vi "main.vi"() -> ()   [LabVIEW 2023]
uses:
  #typedef_state.ctl
  #typedef_action.ctl
  #typedef_data.ctl
panel:
  in  "Mode":dbl(knob) scale=0.0..4.0
  in  "Lid Open 2":bool
  in  "Drying Enable":bool
  in  "Start":bool
  in  "stop":bool
  out "Lid Open":bool
  out "Drying":bool
  out "Centrifugation":bool
  out "Pump watter out":bool
  out "Motor controll":bool
  out "Water heating":bool
  out "Power ON":bool
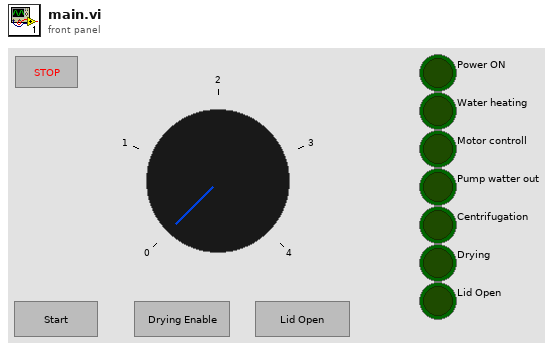
[diagram p1: front panel]
types:
  T1 = typedef "#typedef_state.ctl" = enum16{"Stop", "Drying", "Centrifugation", "Pump watter out", "Motor controll", "Water heating", "Idling", "Inicializing"}
  T2 = typedef "#typedef_action.ctl" = enum16{"pause", "reset", "run"}
  T3 = enum8{"Enabled", "Disabled", "Disabled and Grayed Out"}
  T4 = typedef "#typedef_data.ctl" = cluster{"Power ON":bool, "Water heating":bool, "Motor controll":bool, "Pump watter out":bool, "Centrifugation":bool, "Drying":bool, "Lid Open":bool, "stop":bool, "Start":bool, "Drying Enable":bool, "Lid Open 2":bool, "Mode":dbl, "timereset?":bool}
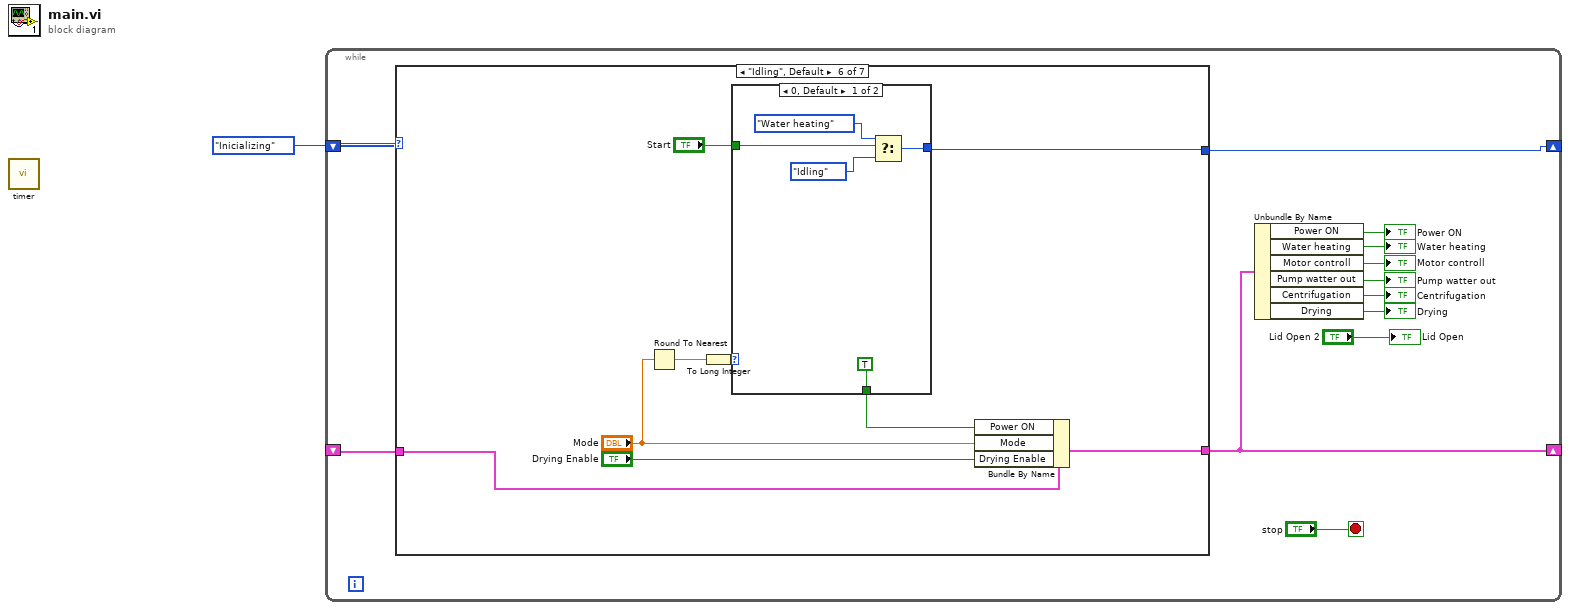
[diagram p0: block diagram]
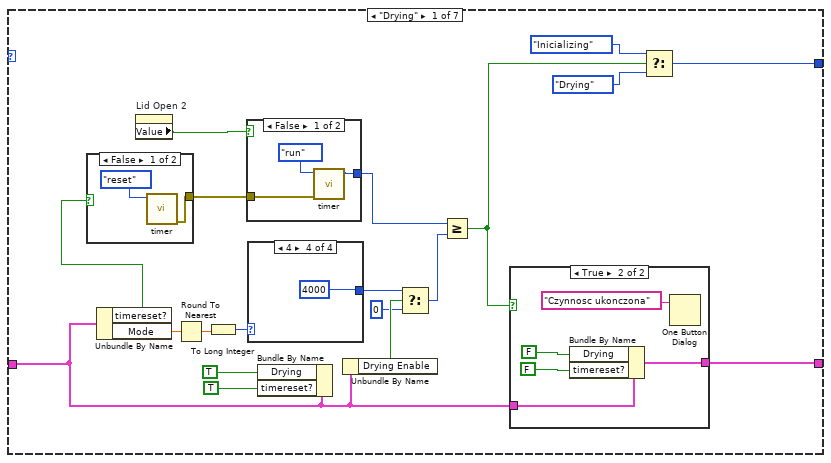
[diagram p2: hidden frame]
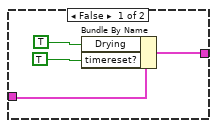
[diagram p3: hidden frame]
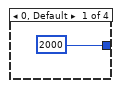
[diagram p4: hidden frame]
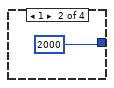
[diagram p5: hidden frame]
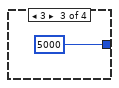
[diagram p6: hidden frame]
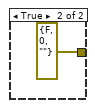
[diagram p7: hidden frame]
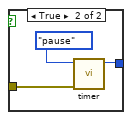
[diagram p8: hidden frame]
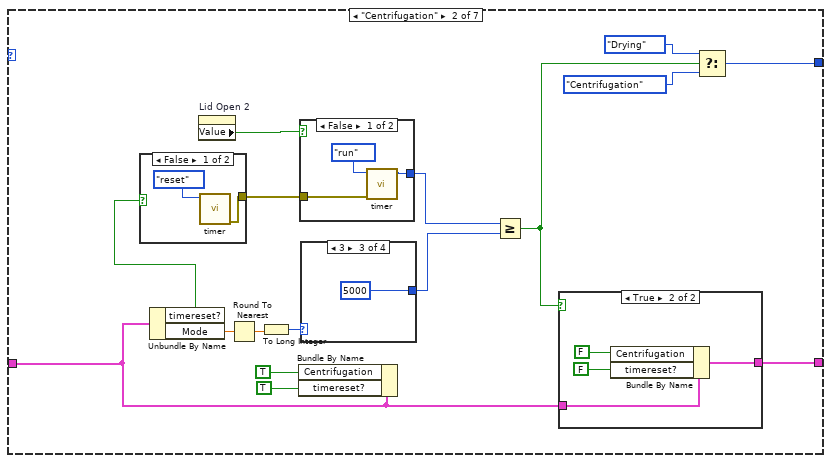
[diagram p9: hidden frame]
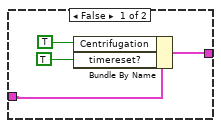
[diagram p10: hidden frame]
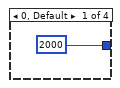
[diagram p11: hidden frame]
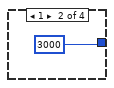
[diagram p12: hidden frame]
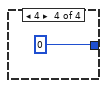
[diagram p13: hidden frame]
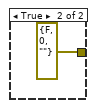
[diagram p14: hidden frame]
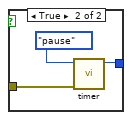
[diagram p15: hidden frame]
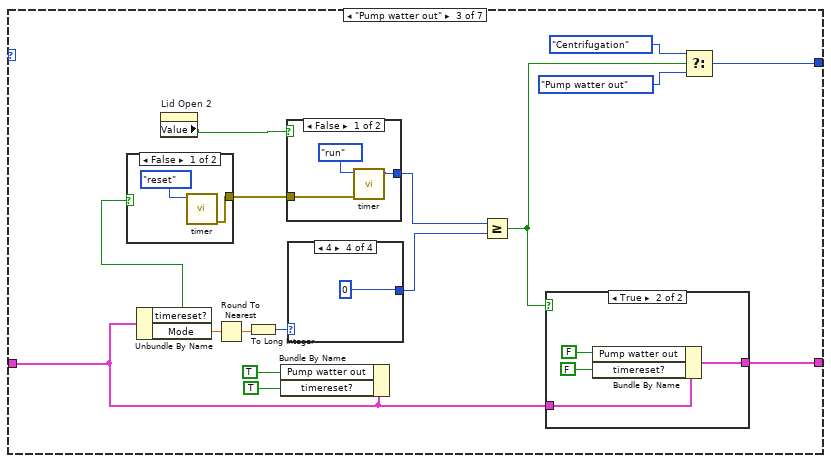
[diagram p16: hidden frame]
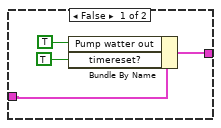
[diagram p17: hidden frame]
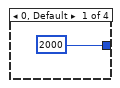
[diagram p18: hidden frame]
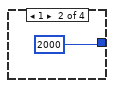
[diagram p19: hidden frame]
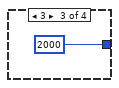
[diagram p20: hidden frame]
diagram:
  n1 = call "timer.vi"() -> ()  [unwired: 10 in, 2 out]
  n2 = while {
    shift-right: [w11] -> _
    shift-left: #typedef_state."Inicializing" ("State") -> [w13]
    shift-right: [w10] -> _
    shift-left: _ -> [w12]
    stop <- "stop" stop-if-true
    n3 = case shown="\"Idling\", Default" w13 {
      tunnel: [w20 w55 w93 w132 w170 w212 T4 {"Power ON"=FALSE, "Water heating"=FALSE, "Motor controll"=FALSE, "Pump watter out"=FALSE, "Centrifugation"=FALSE, "Drying"=FALSE, "Lid Open"=FALSE, "stop"=FALSE, "Start"=FALSE, "Drying Enable"=FALSE, "Lid Open 2"=FALSE, "Mode"=2.05168848812912, "timereset?"=FALSE} ("Data")] -> w10
      tunnel: w12 -> [w18 w56 w94 w131 w171 w213 _]
      tunnel: [w19 w57 w92 w129 w168 w206 #typedef_state."Idling" ("State")] -> w11
      frame "Drying" {
        n4 = Unbundle By Name(w18) -> ("timereset?"=w32:bool, "Mode"=w30:dbl)
        n5 = case shown="False" w32 {
          tunnel: [w46 errorcluster {"status"=FALSE, "code"=0, "source"=""} ("error out")] -> w31
          frame False {
            n6 = call "timer.vi"("Action"=#typedef_action."reset") -> ("error out"=w46:errorcluster)  [unwired: 9 in, 1 out]
          }
          frame True {
          }
        }
        n7 = property on="Lid Open 2" class="Bool (strict)"() -> ("Value"=w21:bool)  [unwired: 2 in, 2 out]
        n8 = Round To Nearest(number=w30) -> (nearest integer value=w26:dbl)
        n9 = To Long Integer(number=w26) -> (32bit integer=w27:i32)
        n10 = case shown="False" w21 {
          tunnel: w31 -> [w51 w53]
          tunnel: [w49 w52] -> w25
          frame False {
            n11 = call "timer.vi"("error in (no error)"=w51, "Action"=#typedef_action."run") -> ("Numeric"=w49:u32)  [unwired: 8 in, 1 out]
          }
          frame True {
            n12 = call "timer.vi"("error in (no error)"=w53, "Action"=#typedef_action."pause") -> ("Numeric"=w52:u32)  [unwired: 8 in, 1 out]
          }
        }
        n13 = case shown="4" w27 {
          tunnel: [2000 2000 5000 4000] -> w15
          frame 0, Default {
          }
          frame 1 {
          }
          frame 3 {
          }
          frame 4 {
          }
        }
        n14 = Bundle By Name(cluster=w18, "Drying"=TRUE ("Water heating"), "timereset?"=TRUE) -> ()  [unwired: 1 out]
        n15 = Unbundle By Name(w18) -> ("Drying Enable"=w17:bool)
        n16 = Select(t=w15, s=w17, f=0) -> (s? t:f=w14:i32)
        n17 = Greater Or Equal?(x=w25, y=w14) -> (x >= y?=w24:bool)
        n18 = case shown="True" w24 {
          tunnel: w18 -> [w33 w39]
          tunnel: [w34 w38] -> w20
          frame False {
            n19 = Bundle By Name(cluster=w33, "Drying"=TRUE ("Water heating"), "timereset?"=TRUE) -> (w34:T4)
          }
          frame True {
            n20 = Bundle By Name(cluster=w39, "Drying"=FALSE ("Water heating"), "timereset?"=FALSE) -> (w38:T4)
            n21 = One Button Dialog(message="Czynnosc ukonczona") -> ()  [unwired: 1 in, 1 out]
          }
        }
        n22 = Select(t=#typedef_state."Inicializing" ("State"), s=w24, f=#typedef_state."Drying") -> (s? t:f=w19:T1)
      }
      frame "Centrifugation" {
        n23 = Unbundle By Name(w56) -> ("timereset?"=w70:bool, "Mode"=w68:dbl)
        n24 = case shown="False" w70 {
          tunnel: [w83 errorcluster {"status"=FALSE, "code"=0, "source"=""} ("error out")] -> w69
          frame False {
            n25 = call "timer.vi"("Action"=#typedef_action."reset") -> ("error out"=w83:errorcluster)  [unwired: 9 in, 1 out]
          }
          frame True {
          }
        }
        n26 = property on="Lid Open 2" class="Bool (strict)"() -> ("Value"=w58:bool)  [unwired: 2 in, 2 out]
        n27 = Round To Nearest(number=w68) -> (nearest integer value=w64:dbl)
        n28 = To Long Integer(number=w64) -> (32bit integer=w65:i32)
        n29 = Bundle By Name(cluster=w56, "Centrifugation"=TRUE ("Water heating"), "timereset?"=TRUE) -> ()  [unwired: 1 out]
        n30 = case shown="False" w58 {
          tunnel: w69 -> [w88 w90]
          tunnel: [w86 w89] -> w63
          frame False {
            n31 = call "timer.vi"("error in (no error)"=w88, "Action"=#typedef_action."run") -> ("Numeric"=w86:u32)  [unwired: 8 in, 1 out]
          }
          frame True {
            n32 = call "timer.vi"("error in (no error)"=w90, "Action"=#typedef_action."pause") -> ("Numeric"=w89:u32)  [unwired: 8 in, 1 out]
          }
        }
        n33 = case shown="3" w65 {
          tunnel: [2000 3000 5000 0] -> w62
          frame 0, Default {
          }
          frame 1 {
          }
          frame 3 {
          }
          frame 4 {
          }
        }
        n34 = Greater Or Equal?(x=w63, y=w62) -> (x >= y?=w61:bool)
        n35 = case shown="True" w61 {
          tunnel: w56 -> [w71 w76]
          tunnel: [w72 w75] -> w55
          frame False {
            n36 = Bundle By Name(cluster=w71, "Centrifugation"=TRUE ("Water heating"), "timereset?"=TRUE) -> (w72:T4)
          }
          frame True {
            n37 = Bundle By Name(cluster=w76, "Centrifugation"=FALSE ("Water heating"), "timereset?"=FALSE) -> (w75:T4)
          }
        }
        n38 = Select(t=#typedef_state."Drying" ("State"), s=w61, f=#typedef_state."Centrifugation") -> (s? t:f=w57:T1)
      }
      frame "Pump watter out" {
        n39 = Unbundle By Name(w94) -> ("timereset?"=w107:bool, "Mode"=w105:dbl)
        n40 = case shown="False" w107 {
          tunnel: [w120 errorcluster {"status"=FALSE, "code"=0, "source"=""} ("error out")] -> w106
          frame False {
            n41 = call "timer.vi"("Action"=#typedef_action."reset") -> ("error out"=w120:errorcluster)  [unwired: 9 in, 1 out]
          }
          frame True {
          }
        }
        n42 = property on="Lid Open 2" class="Bool (strict)"() -> ("Value"=w95:bool)  [unwired: 2 in, 2 out]
        n43 = Round To Nearest(number=w105) -> (nearest integer value=w101:dbl)
        n44 = To Long Integer(number=w101) -> (32bit integer=w102:i32)
        n45 = Bundle By Name(cluster=w94, "Pump watter out"=TRUE ("Water heating"), "timereset?"=TRUE) -> ()  [unwired: 1 out]
        n46 = case shown="False" w95 {
          tunnel: w106 -> [w125 w127]
          tunnel: [w123 w126] -> w100
          frame False {
            n47 = call "timer.vi"("error in (no error)"=w125, "Action"=#typedef_action."run") -> ("Numeric"=w123:u32)  [unwired: 8 in, 1 out]
          }
          frame True {
            n48 = call "timer.vi"("error in (no error)"=w127, "Action"=#typedef_action."pause") -> ("Numeric"=w126:u32)  [unwired: 8 in, 1 out]
          }
        }
        n49 = case shown="4" w102 {
          tunnel: [2000 2000 2000 0] -> w99
          frame 0, Default {
          }
          frame 1 {
          }
          frame 3 {
          }
          frame 4 {
          }
        }
        n50 = Greater Or Equal?(x=w100, y=w99) -> (x >= y?=w98:bool)
        n51 = case shown="True" w98 {
          tunnel: w94 -> [w108 w113]
          tunnel: [w109 w112] -> w93
          frame False {
            n52 = Bundle By Name(cluster=w108, "Pump watter out"=TRUE ("Water heating"), "timereset?"=TRUE) -> (w109:T4)
          }
          frame True {
            n53 = Bundle By Name(cluster=w113, "Pump watter out"=FALSE ("Water heating"), "timereset?"=FALSE) -> (w112:T4)
          }
        }
        n54 = Select(t=#typedef_state."Centrifugation" ("State"), s=w98, f=#typedef_state."Pump watter out") -> (s? t:f=w92:T1)
      }
      frame "Motor controll" {
        n55 = Unbundle By Name(w131) -> ("timereset?"=w144:bool, "Mode"=w142:dbl)
        n56 = case shown="False" w144 {
          tunnel: [w157 errorcluster {"status"=FALSE, "code"=0, "source"=""} ("error out")] -> w143
          frame False {
            n57 = call "timer.vi"("Action"=#typedef_action."reset") -> ("error out"=w157:errorcluster)  [unwired: 9 in, 1 out]
          }
          frame True {
          }
        }
        n58 = property on="Lid Open 2" class="Bool (strict)"() -> ("Value"=w130:bool)  [unwired: 2 in, 2 out]
        n59 = Round To Nearest(number=w142) -> (nearest integer value=w138:dbl)
        n60 = To Long Integer(number=w138) -> (32bit integer=w139:i32)
        n61 = case shown="False" w130 {
          tunnel: w143 -> [w162 w164]
          tunnel: [w160 w163] -> w137
          frame False {
            n62 = call "timer.vi"("error in (no error)"=w162, "Action"=#typedef_action."run") -> ("Numeric"=w160:u32)  [unwired: 8 in, 1 out]
          }
          frame True {
            n63 = call "timer.vi"("error in (no error)"=w164, "Action"=#typedef_action."pause") -> ("Numeric"=w163:u32)  [unwired: 8 in, 1 out]
          }
        }
        n64 = Bundle By Name(cluster=w131, "Motor controll"=TRUE ("Water heating"), "timereset?"=TRUE) -> ()  [unwired: 1 out]
        n65 = case shown="3" w139 {
          tunnel: [2000 4000 6000 0] -> w136
          frame 0, Default {
          }
          frame 1 {
          }
          frame 3 {
          }
          frame 4 {
          }
        }
        n66 = Greater Or Equal?(x=w137, y=w136) -> (x >= y?=w135:bool)
        n67 = case shown="True" w135 {
          tunnel: w131 -> [w145 w150]
          tunnel: [w146 w149] -> w132
          frame False {
            n68 = Bundle By Name(cluster=w145, "Motor controll"=TRUE ("Water heating"), "timereset?"=TRUE) -> (w146:T4)
          }
          frame True {
            n69 = Bundle By Name(cluster=w150, "Motor controll"=FALSE ("Water heating"), "timereset?"=FALSE) -> (w149:T4)
          }
        }
        n70 = Select(t=#typedef_state."Pump watter out" ("State"), s=w135, f=#typedef_state."Motor controll") -> (s? t:f=w129:T1)
      }
      frame "Water heating" {
        n71 = Unbundle By Name(w171) -> ("timereset?"=w181:bool, "Mode"=w179:dbl)
        n72 = case shown="False" w181 {
          tunnel: [w196 errorcluster {"status"=FALSE, "code"=0, "source"=""} ("error out")] -> w180
          frame False {
            n73 = call "timer.vi"("Action"=#typedef_action."reset") -> ("error out"=w196:errorcluster)  [unwired: 9 in, 1 out]
          }
          frame True {
          }
        }
        n74 = property on="Mode" class="Knob (strict)"("DisabledEnum"=T3."Disabled" ("Disabled")) -> ()  [unwired: 2 in, 2 out]
        n75 = property on="Drying Enable" class="Bool (strict)"("DisabledEnum"=T3."Disabled" ("Disabled")) -> ()  [unwired: 2 in, 2 out]
        n76 = property on="Lid Open 2" class="Bool (strict)"() -> ("Value"=w166:bool)  [unwired: 2 in, 2 out]
        n77 = Round To Nearest(number=w179) -> (nearest integer value=w175:dbl)
        n78 = To Long Integer(number=w175) -> (32bit integer=w176:i32)
        n79 = case shown="False" w166 {
          tunnel: w180 -> [w201 w203]
          tunnel: [w199 w202] -> w174
          frame False {
            n80 = call "timer.vi"("error in (no error)"=w201, "Action"=#typedef_action."run") -> ("Numeric"=w199:u32)  [unwired: 8 in, 1 out]
          }
          frame True {
            n81 = call "timer.vi"("error in (no error)"=w203, "Action"=#typedef_action."pause") -> ("Numeric"=w202:u32)  [unwired: 8 in, 1 out]
          }
        }
        n82 = Bundle By Name(cluster=w171, "Water heating"=TRUE, "timereset?"=TRUE) -> ()  [unwired: 1 out]
        n83 = case shown="4" w176 {
          tunnel: [2000 3000 4000 0] -> w173
          frame 0, Default {
          }
          frame 1 {
          }
          frame 3 {
          }
          frame 4 {
          }
        }
        n84 = Greater Or Equal?(x=w174, y=w173) -> (x >= y?=w172:bool)
        n85 = case shown="False" w172 {
          tunnel: w171 -> [w184 w189]
          tunnel: [w185 w188] -> w170
          frame False {
            n86 = Bundle By Name(cluster=w184, "Water heating"=TRUE, "timereset?"=TRUE) -> (w185:T4)
          }
          frame True {
            n87 = Bundle By Name(cluster=w189, "Water heating"=FALSE, "timereset?"=FALSE) -> (w188:T4)
          }
        }
        n88 = Select(t=#typedef_state."Motor controll" ("State"), s=w172, f=#typedef_state."Water heating") -> (s? t:f=w168:T1)
      }
      frame "Idling", Default {
        n89 = Round To Nearest(number="Mode") -> (nearest integer value=w208:dbl)
        n90 = To Long Integer(number=w208) -> (32bit integer=w209:i32)
        n91 = case shown="0, Default" w209 {
          tunnel: [TRUE FALSE] -> w207
          tunnel: [w215 #typedef_state."Idling" ("State")] -> w206
          tunnel: "Start" -> [w214 _]
          frame 0, Default {
            n92 = Select(t=#typedef_state."Water heating", s=w214, f=#typedef_state."Idling" ("State")) -> (s? t:f=w215:T1)
          }
          frame 2 {
          }
        }
        n93 = Bundle By Name(cluster=w213, "Power ON"=w207, "Mode"="Mode", "Drying Enable"="Drying Enable") -> (w212:T4)
      }
      frame "Inicializing" {
        n94 = property on="Mode" class="Knob (strict)"("DisabledEnum"=T3."Enabled" ("Disabled")) -> ()  [unwired: 2 in, 2 out]
        n95 = property on="Drying Enable" class="Bool (strict)"("DisabledEnum"=T3."Enabled" ("Disabled")) -> ()  [unwired: 2 in, 2 out]
      }
    }
    n96 = Unbundle By Name(w10) -> ("Power ON"=→"Power ON":bool, "Water heating"=→"Water heating":bool, "Motor controll"=→"Motor controll":bool, "Pump watter out"=→"Pump watter out":bool, "Centrifugation"=→"Centrifugation":bool, "Drying"=→"Drying":bool)
    "Lid Open" <- "Lid Open 2"
  }
